vi "Generate DGML footer.vi"() -> (0 "string":string)   [LabVIEW 2018, in "DGML creation.lvlib"]
uses:
  DGML creation.lvlib
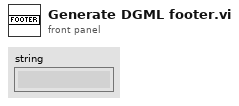
[diagram p1: front panel]
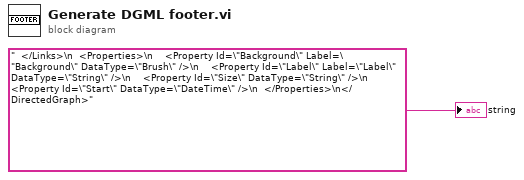
[diagram p0: block diagram]
diagram:
  "string" <- "  </Links>\n  <Properties>\n    <Property Id=\"Background\" Label=\"Background\" DataType=\"Brush\" />\n    <Property Id=\"Label\" Label=\"Label\" DataType=\"String\" />\n    <Property Id=\"Size\" DataType=\"String\" />\n    <Property Id=\"Start\" DataType=\"DateTime\" />\n  </Properties>\n</DirectedGraph>" ("string")
